vi "SendCommand.vi"(2 "timeout ms":i32=-1, 3 "command":string) -> (0 "reply":string="\r\n", 1 "Error":bool)   [LabVIEW 2014]
uses:
  globals/AzCamGlobals.vi
panel:
  out "error out":errorcluster
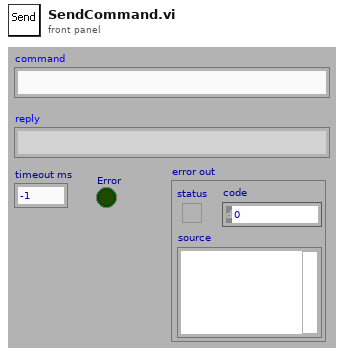
[diagram p1: front panel]
types:
  T1 = enum16{"Standard", "Buffered", "CRLF", "Immediate"}
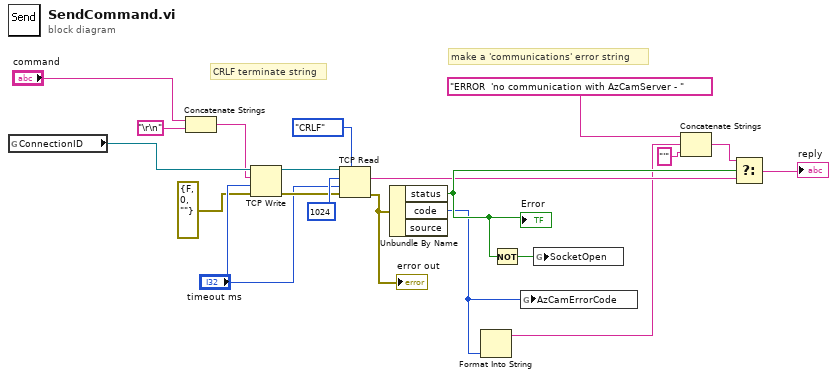
[diagram p0: block diagram]
diagram:
  # "make a 'communications' error string"
  # "CRLF terminate string"
  n1 = global read "AzCamGlobals.vi" "ConnectionID"() -> (w12:refnum<k5>)
  n2 = Concatenate Strings("command", "\r\n") -> (w10:string)
  n3 = TCP Write(connection ID=w12, data in=w10, error in (no error)=errorcluster {"status"=FALSE, "code"=0, "source"=""}, 9:"timeout ms") -> (connection ID out=w17:refnum<k5>, error out=w15:errorcluster)  [unwired: 1 out]
  n4 = TCP Read(connection ID=w17, bytes to read=1024, error in (no error)=w15, 7:T1."CRLF" ("mode (standard)"), 9:"timeout ms") -> (data out=w8:string, error out=w7:errorcluster)  [unwired: 1 out]
  "error out" <- w7
  n5 = Unbundle By Name(w7) -> ("status"=w18:bool, "code"=w5:i32)  [unwired: 1 out]
  "Error" <- w18
  n6 = Format Into String(w5) -> (resulting string=w4:string)  [unwired: 3 in, 1 out]
  n7 = Not(x=w18) -> (.not. x?=w9:bool)
  n8 = global write "AzCamGlobals.vi" "AzCamErrorCode"(w5) -> ()
  n9 = global write "AzCamGlobals.vi" "SocketOpen"(w9) -> ()
  n10 = Concatenate Strings("ERROR  'no communication with AzCamServer - " ("data out"), w4, "'" ("string")) -> (w1:string)
  n11 = Select(t=w1, s=w18, f=w8) -> (s? t:f=→"reply":string)
